vi "configuration UI.vi"() -> ()   [LabVIEW 2013, in "tag bus configurable plugin editor node.lvclass"]
uses:
  tag bus configurable plugin editor node.lvclass
  <vilib>/NI/Configuration Framework/Node/NodeRef.ctl
  <vilib>/NI/Configuration Framework/Node/NISE_CEF_Node.lvclass
  <vilib>/NI/AMC/Message Queue.ctl
  <vilib>/NI/AMC/Message.ctl
  <vilib>/NI/Tools/Keyed Array/KeyedArray.ctl
  <vilib>/NI/Configuration Framework/Node/UserEventRef.ctl
  <vilib>/NI/Configuration Framework/Controls/EventCluster.ctl
  <vilib>/NI/DCAF UI Toolkit/Controls/Configure.ctl
  <vilib>/NI/DCAF UI Toolkit/Controls/Add.ctl
  <vilib>/NI/DCAF UI Toolkit/Controls/Remove.ctl
  <vilib>/NI/Configuration Framework/Node/StopEvent.ctl
  <vilib>/NI/Configuration Framework/Node/RefreshUIEvent.ctl
  <vilib>/NI/Configuration Framework/Node/CacheState.ctl
  <vilib>/NI/Configuration Framework/Node/NodeChangeEvent.ctl
  <vilib>/NI/Tag Bus/tag/Data Type.ctl
  Permissions Enum.ctl
  Available Tag Menu/channel action event.ctl
  Available Tag Menu/dialog output action.ctl
  <vilib>/NI/Tag Bus Module Framework/channel/TBM channel.lvclass
  <vilib>/NI/Tag Bus/tag/tag descriptor.lvclass
  Table Manager/Call Back Ref Type Def.ctl
  Configuration Editor/Classes/Engine Parent/Engine Parent Editor Node.lvclass
  Configuration Editor/Classes/Module editor node/module editor node.lvclass
  Listbox/Multi Column Listbox.lvclass
  <vilib>/NI/Configuration Framework/NISE_CEF_TreeControl.lvlib
  <vilib>/NI/Tools/Keyed Array/Tools_KeyedArray.lvlib
  <vilib>/NI/AMC/AMC.lvlib
  Table Manager.lvlib
  Table Manager/references.ctl
  Table Manager/Table Manager.lvclass
  testing/Table Manager tests.lvlib
  <vilib>/NI/DCAF UI Toolkit/Controls/DCAF UI Elements.lvlib
panel:
  in  "user event out":refnum<user-event>
  in  "Permissions":T1
  in  "data type":T2
  in  "node change":T3
  in  "cache state":T4
  in  "refresh UI":T5
  in  "stop event":T6
  in  "Tab Control":enum32{"Static Configuration"}(tab)
  in  "Remove Button":T7
  in  "Add Button":T8
  in  "Table":i32(listbox)
  in  "settings":T9
  in  "user event":T10
  in  "main queue":T11
  in  "node ref":T12
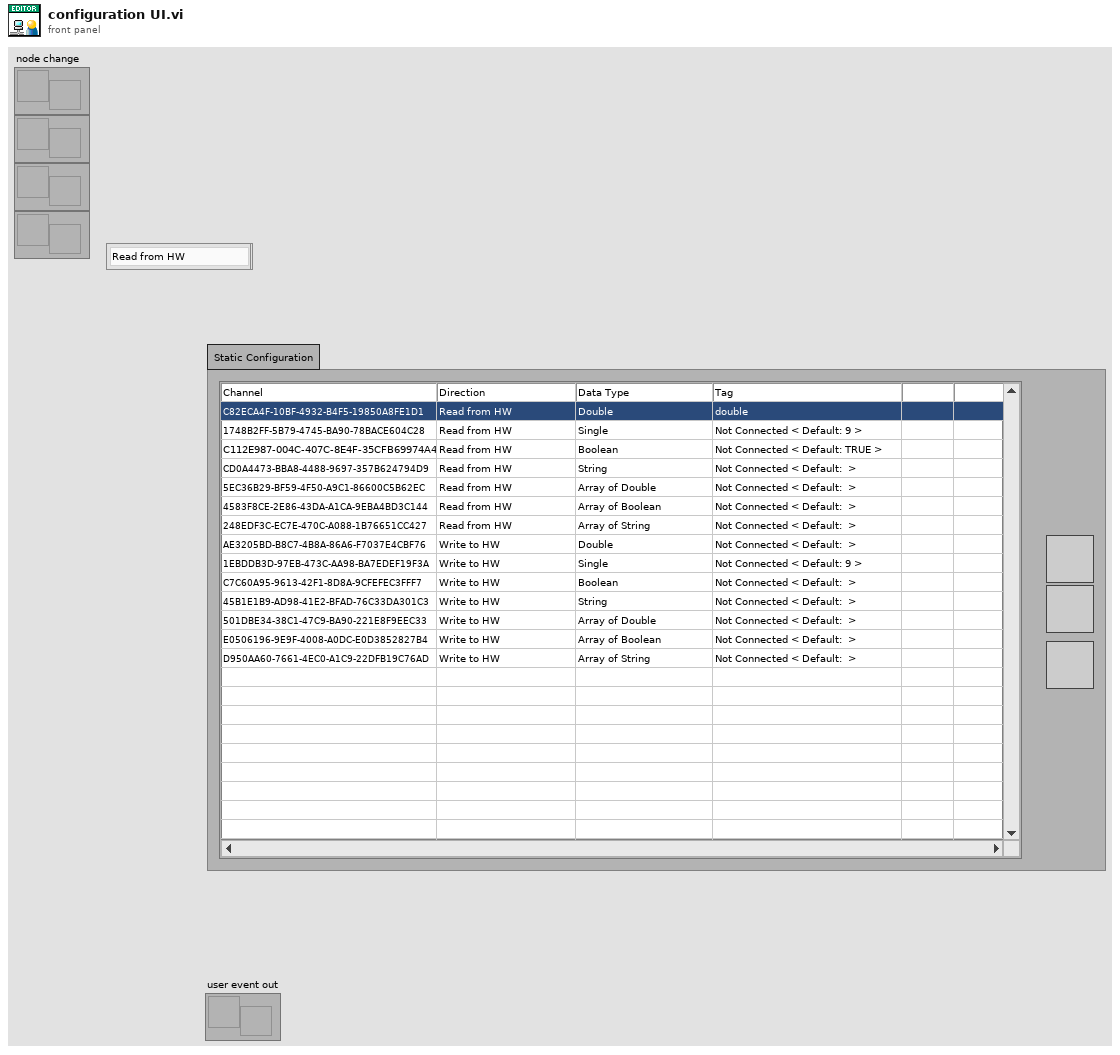
[diagram p1: front panel]
types:
  T1 = typedef "tag bus configurable plugin editor node.lvclass/Permissions Enum.ctl" = enum16{"Read from HW", "Write to HW"}
  T2 = typedef "tag bus.lvlib/tag descriptor.lvclass/Data Type.ctl" = enum16{"Double", "Single", "I64", "I32", "I16", "I8", "U64", "U32", "U16", "U8", "Boolean", "String", "Array of Double", "Array of Single", "Array of I64", "Array of I32", "Array of I16", "Array of I8", "Array of U64", "Array of U32", "Array of U16", "Array of U8", "Array of Boolean", "Array of String"}
  T3 = typedef "NISE_CEF_Node.lvclass/NodeChangeEvent.ctl" = refnum<user-event>
  T4 = typedef "NISE_CEF_Node.lvclass/CacheState.ctl" = refnum<user-event>
  T5 = typedef "NISE_CEF_Node.lvclass/RefreshUIEvent.ctl" = refnum<user-event>
  T6 = typedef "NISE_CEF_Node.lvclass/StopEvent.ctl" = refnum<user-event>
  T7 = typedef "DCAF UI Elements.lvlib/Remove.ctl" = bool
  T8 = typedef "DCAF UI Elements.lvlib/Add.ctl" = bool
  T9 = typedef "DCAF UI Elements.lvlib/Configure.ctl" = bool
  T10 = typedef "NISE_CEF_Node.lvclass/UserEventRef.ctl" = refnum<user-event>
  T11 = typedef "AMC.lvlib/Message Queue.ctl" = refnum<queue>
  T12 = typedef "NISE_CEF_Node.lvclass/NodeRef.ctl" = refnum<data-value>
  T13 = typedef "Table Manager.lvlib/Table Manager.lvclass/references.ctl" = cluster{"stop event":T6, "refresh UI":T5, "cache state":T4, "node change":T3, "user event out":refnum<user-event>, "main queue":T11, "user event":T10}
  T14 = typedef "Table Manager.lvlib/Table Manager.lvclass/object ref.ctl" = cluster{"engine":refnum<data-value>, "Node Ref":refnum<data-value>}
  T15 = typedef "Table Manager.lvlib/Column.lvclass/Column Descriptor.ctl" = cluster{"name":string, "caption":string, "Column Type":T16, "Params":string, "AutoSizeMode":i32, "FillWeight":sgl, "MinWidth":u32, "tooltip":string, "Enum Reference":refnum<vi>, "Channel suffix":string, "Read Only":bool, "Call Back VI":T17, "DT Dependency":i32, "name dependency":i32, "data type":T2, "Custom Column":refnum<class "Column.lvclass">}
  T16 = typedef "Table Manager.lvlib/Column.lvclass/Column Type.ctl" = enum16{"String", "Mapping", "Enum", "Custom"}
  T17 = typedef "Table Manager.lvlib/Table Manager.lvclass/Call Back Ref Type Def.ctl" = refnum<vi>
  T18 = typedef "Table Manager.lvlib/Table Manager.lvclass/Table Events.ctl" = cluster{"Menu Selection":refnum<user-event>}
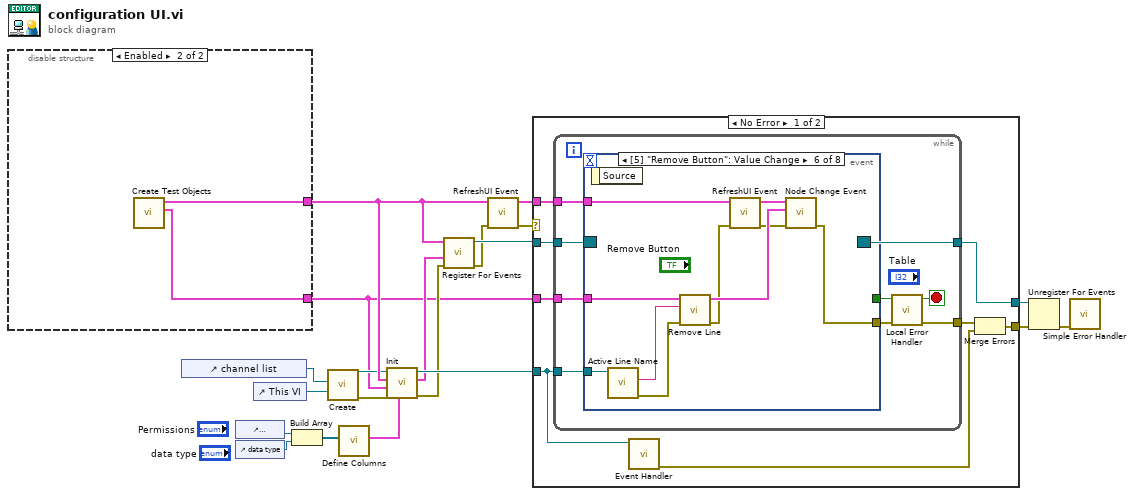
[diagram p0: block diagram]
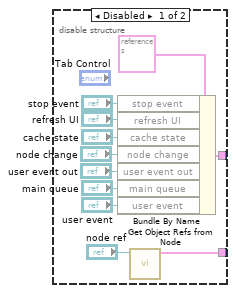
[diagram p2: hidden frame]
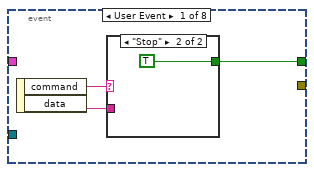
[diagram p3: hidden frame]
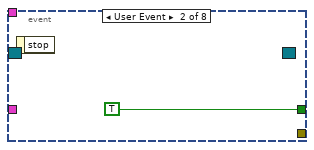
[diagram p5: hidden frame]
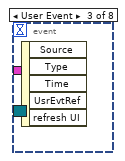
[diagram p6: hidden frame]
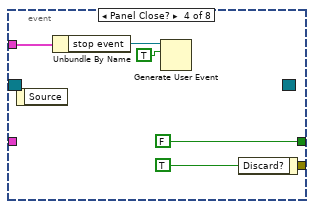
[diagram p7: hidden frame]
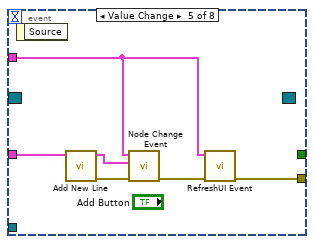
[diagram p8: hidden frame]
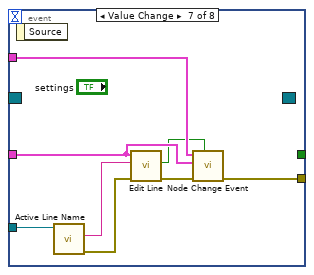
[diagram p9: hidden frame]
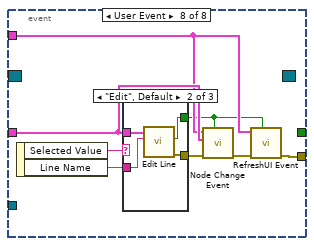
[diagram p10: hidden frame]
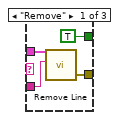
[diagram p11: hidden frame]
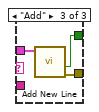
[diagram p12: hidden frame]
diagram:
  n1 = disable-structure shown="Enabled" {
    disable-tunnel: [w24 w32] -> w1
    disable-tunnel: [w21 w33] -> w7
    frame Disabled {
      n2 = Bundle By Name(cluster=T13 {"stop event"=refnum, "refresh UI"=refnum, "cache state"=refnum, "node change"=refnum, "user event out"=refnum, "main queue"=refnum, "user event"=refnum} ("References"), "stop event"="stop event", "refresh UI"="refresh UI", "cache state"="cache state", "node change"="node change", "user event out"="user event out", "main queue"="main queue", "user event"="user event") -> (w21:T13)
      n3 = call "Get Object Refs from Node.vi"("Data Value Reference in"="node ref") -> ("references"=w24:T14)  [unwired: 9 in, 1 out]
    }
    frame Enabled {
      n4 = call "Create Test Objects.vi"() -> ("Objects"=w32:T14, "Refs"=w33:T13)  [unwired: 7 in, 3 out]
    }
  }
  n5 = control-ref of="channel list"() -> (w5:refnum<vi>)
  n6 = control-ref of="Permissions"() -> (w14:refnum<vi>)
  n7 = control-ref of="data type"() -> (w13:refnum<vi>)
  n8 = control-ref of="This VI"() -> (w4:refnum<vi>)
  n9 = Build Array(w14, w13) -> (w12:refnum<vi>[])
  n10 = call "Create.vi"("Top VI"=w4, "Listbox"=w5) -> ("error out"=w3:errorcluster, "reference out"=w2:refnum<class "Multi Column Listbox.lvclass">)  [unwired: 8 in]
  n11 = call "Define Columns.vi"("Enum Array"=w12) -> ("Column Definition"=w16:T15[])  [unwired: 10 in]
  n12 = call-dynamic "Init.vi"("Column Descriptors"=w16, "error in (no error)"=w3, "Node object refs"=w1, "Event References"=w7, "Multi Column Listbox in"=w2) -> ("error out"=w8:errorcluster, "Table Events"=w6:T18, "Multi Column Listbox out"=w11:refnum<class "Multi Column Listbox.lvclass">)  [unwired: 4 in]
  n13 = call "Register For Events.vi"("error in"=w8, "Table Events"=w6, "References"=w7) -> ("error out"=w10:errorcluster, "Event Registration Refnum"=w17:refnum<event-registration>)  [unwired: 7 in]
  n14 = call "RefreshUI Event.vi"("error in (no error)"=w10, "References in"=w7) -> ("error out"=w9:errorcluster, "References out"=w15:T13)  [unwired: 8 in]
  n15 = case shown="No Error" w9 {
    selector: w9 -> [_ w103]
    tunnel: w17 -> [w41 w102]
    tunnel: [w40 w102] -> w20
    tunnel: [w34 w103] -> w19
    tunnel: w15 -> [w39 _]
    tunnel: w1 -> [w38 _]
    tunnel: w11 -> [w37 _]
    frame No Error {
      n16 = while {
        tunnel: w41 -> [w50]
        tunnel: [w49] -> w40
        tunnel: [w46] -> w35
        tunnel: w39 -> [w44]
        tunnel: w38 -> [w43]
        tunnel: w37 -> [w42]
        stop <- w48 stop-if-true
        n17 = event shown="[5] \"Remove Button\": Value Change" {
          selector: w50 -> [_ _ _ _ _ _ _ _]
          dyn-events: [_ _ _ _ _ _ _ _] -> w49
          timeout: _ -> [_ _ _ _ _ _ _ _]
          tunnel: [w53 TRUE _ FALSE _ _ _ _] -> w47
          tunnel: [_ _ _ _ w61 w69 w80 w87] -> w45
          tunnel: w44 -> [_ _ _ w57 w64 w74 w82 w84]
          tunnel: w43 -> [_ _ _ _ w65 w73 w78 w85]
          tunnel: w42 -> [_ _ _ _ _ w68 w79 _]
          event User Event {
            n18 = event-data() -> ("command"=w52:string, "data"=w51:string)  [unwired: 1 in]
            n19 = case shown="\"Stop\"" w52 {
              tunnel: [_ TRUE] -> w53
              tunnel: w51 -> [_ _]
              frame Default {
              }
              frame "Stop" {
              }
            }
          }
          event User Event {
            n20 = event-data() -> ()  [unwired: 1 in, 1 out]
          }
          event User Event {
            n21 = event-data() -> ()  [unwired: 1 in, 5 out]
          }
          event Panel Close? {
            n22 = event-data() -> ()  [unwired: 1 in, 1 out]
            n23 = Unbundle By Name(w57) -> ("stop event"=w56:T6)
            n24 = Generate User Event(user event=w56, event data cluster=TRUE ("event data")) -> ()  [unwired: 2 in, 2 out]
            n25 = event-data("Discard?"=TRUE) -> ()  [unwired: 1 in, 1 out]
          }
          event Value Change {
            n26 = event-data() -> ()  [unwired: 1 in, 1 out]
            n27 = call "Add New Line.vi"("objects"=w65) -> ("error out"=w63:errorcluster)  [unwired: 9 in, 1 out]
            n28 = call "Node Change Event.vi"("error in (no error)"=w63, "objects"=w65, "References in"=w64) -> ("error out"=w62:errorcluster)  [unwired: 8 in]
            n29 = call "RefreshUI Event.vi"("error in (no error)"=w62, "References in"=w64) -> ("error out"=w61:errorcluster)  [unwired: 8 in, 1 out]
          }
          event Value Change {
            n30 = event-data() -> ()  [unwired: 1 in, 1 out]
            n31 = call-dynamic "Active Line Name.vi"("Multi Column Listbox in"=w68) -> ("error out"=w66:errorcluster, "Active Line Name"=w67:string)  [unwired: 8 in, 1 out]
            n32 = call "Remove Line.vi"("error in"=w66, "Active Line Name"=w67, "Objects"=w73) -> ("error out"=w70:errorcluster)  [unwired: 8 in]
            n33 = call "RefreshUI Event.vi"("error in (no error)"=w70, "References in"=w74) -> ("error out"=w72:errorcluster, "References out"=w71:T13)  [unwired: 8 in]
            n34 = call "Node Change Event.vi"("error in (no error)"=w72, "objects"=w73, "References in"=w71) -> ("error out"=w69:errorcluster)  [unwired: 8 in]
          }
          event Value Change {
            n35 = event-data() -> ()  [unwired: 1 in, 1 out]
            n36 = call-dynamic "Active Line Name.vi"("Multi Column Listbox in"=w79) -> ("error out"=w76:errorcluster, "Active Line Name"=w77:string)  [unwired: 8 in, 1 out]
            n37 = call "Edit Line.vi"("error in"=w76, "Line Name"=w77, "References"=w78) -> ("error out"=w81:errorcluster, "change?"=w75:bool)  [unwired: 7 in]
            n38 = call "Node Change Event.vi"("Send"=w75, "error in (no error)"=w81, "objects"=w78, "References in"=w82) -> ("error out"=w80:errorcluster)  [unwired: 7 in]
          }
          event User Event {
            n39 = event-data() -> ("Selected Value"=w90:string, "Line Name"=w89:string)  [unwired: 1 in]
            n40 = case shown="\"Edit\", Default" w90 {
              tunnel: w85 -> [w94 w97 w101]
              tunnel: w89 -> [w93 w98 _]
              tunnel: [w92 w96 w100] -> w86
              tunnel: [TRUE ("success") w95 w99] -> w83
              frame "Remove" {
                n41 = call "Remove Line.vi"("Active Line Name"=w93, "Objects"=w94) -> ("error out"=w92:errorcluster)  [unwired: 9 in]
              }
              frame "Edit", Default {
                n42 = call "Edit Line.vi"("Line Name"=w98, "References"=w97) -> ("error out"=w96:errorcluster, "change?"=w95:bool)  [unwired: 8 in]
              }
              frame "Add" {
                n43 = call "Add New Line.vi"("objects"=w101) -> ("error out"=w100:errorcluster, "success"=w99:bool)  [unwired: 9 in]
              }
            }
            n44 = call "Node Change Event.vi"("Send"=w83, "error in (no error)"=w86, "objects"=w85, "References in"=w84) -> ("error out"=w88:errorcluster)  [unwired: 7 in]
            n45 = call "RefreshUI Event.vi"("Refresh"=w83, "error in (no error)"=w88, "References in"=w84) -> ("error out"=w87:errorcluster)  [unwired: 7 in, 1 out]
          }
        }
        n46 = call "Local Error Handler.vi"("error in"=w45, "Stop in"=w47) -> ("error out"=w46:errorcluster, "Stop out"=w48:bool)  [unwired: 8 in]
      }
      n47 = call-dynamic "Event Handler.vi"("Listbox in"=w37) -> ("error out"=w36:errorcluster)  [unwired: 9 in, 1 out]
      n48 = Merge Errors(w35, w36) -> (w34:errorcluster)
    }
    frame Error {
    }
  }
  n49 = Unregister For Events(event registration refnum=w20, error in=w19) -> (error out=w18:errorcluster)
  n50 = call <vilib>:"Simple Error Handler.vi"("error in (no error)"=w18) -> ()  [unwired: 4 in, 5 out]
